vi "TD VI.vi"() -> ()   [LabVIEW 2016]
panel:
  out "Desvio Padrão":dbl
  out "Média":dbl
  out "Vetor de amostras":dbl[](array[numeric])
  out "Waveform Chart":dbl(graph)
  out "Amostra":dbl
  out "error out":errorcluster
  in  "acende botão":bool
  in  "Stop Button":bool
  in  "Send":bool
  in  "VISA resource name":refnum<visa-resource-name>
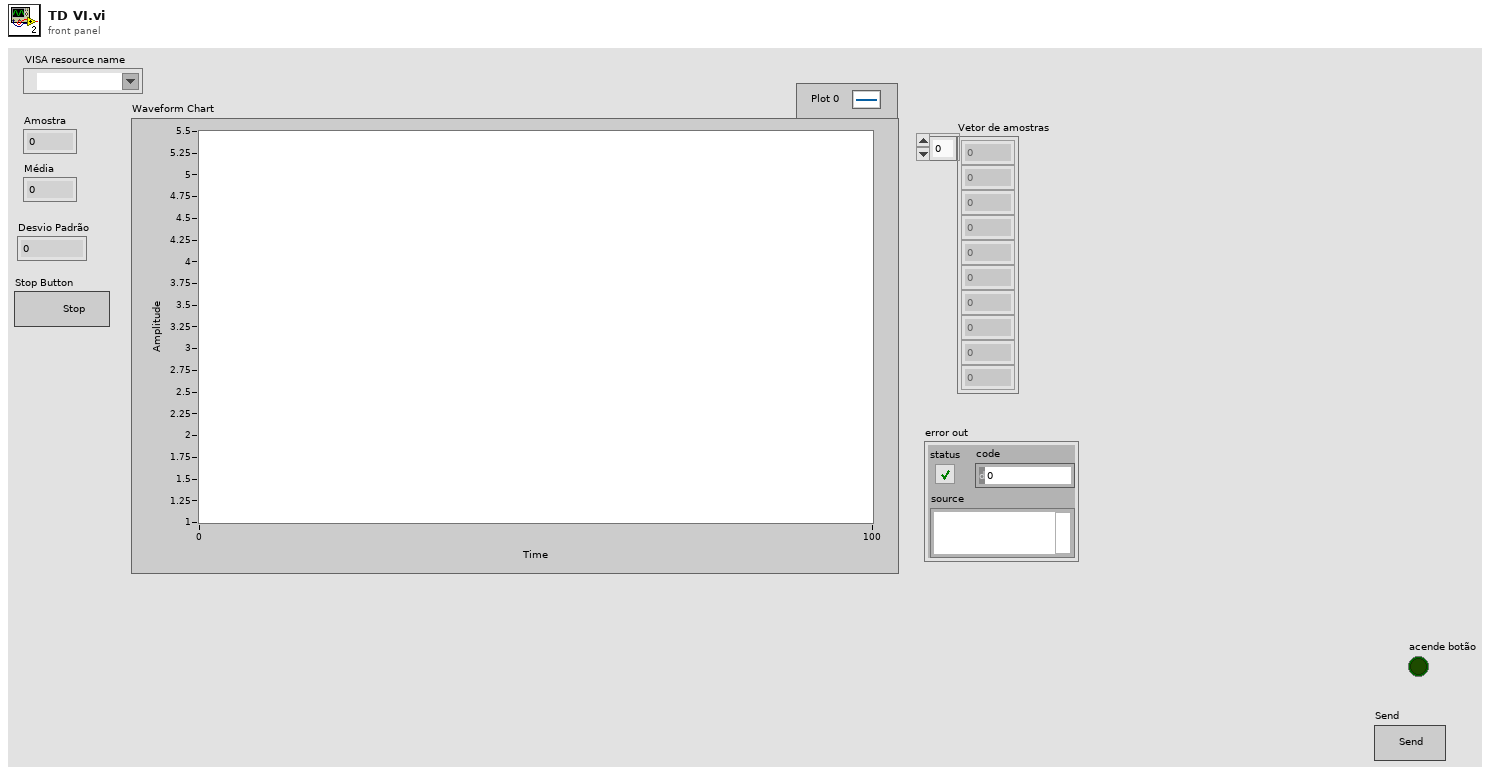
[diagram p1: front panel]
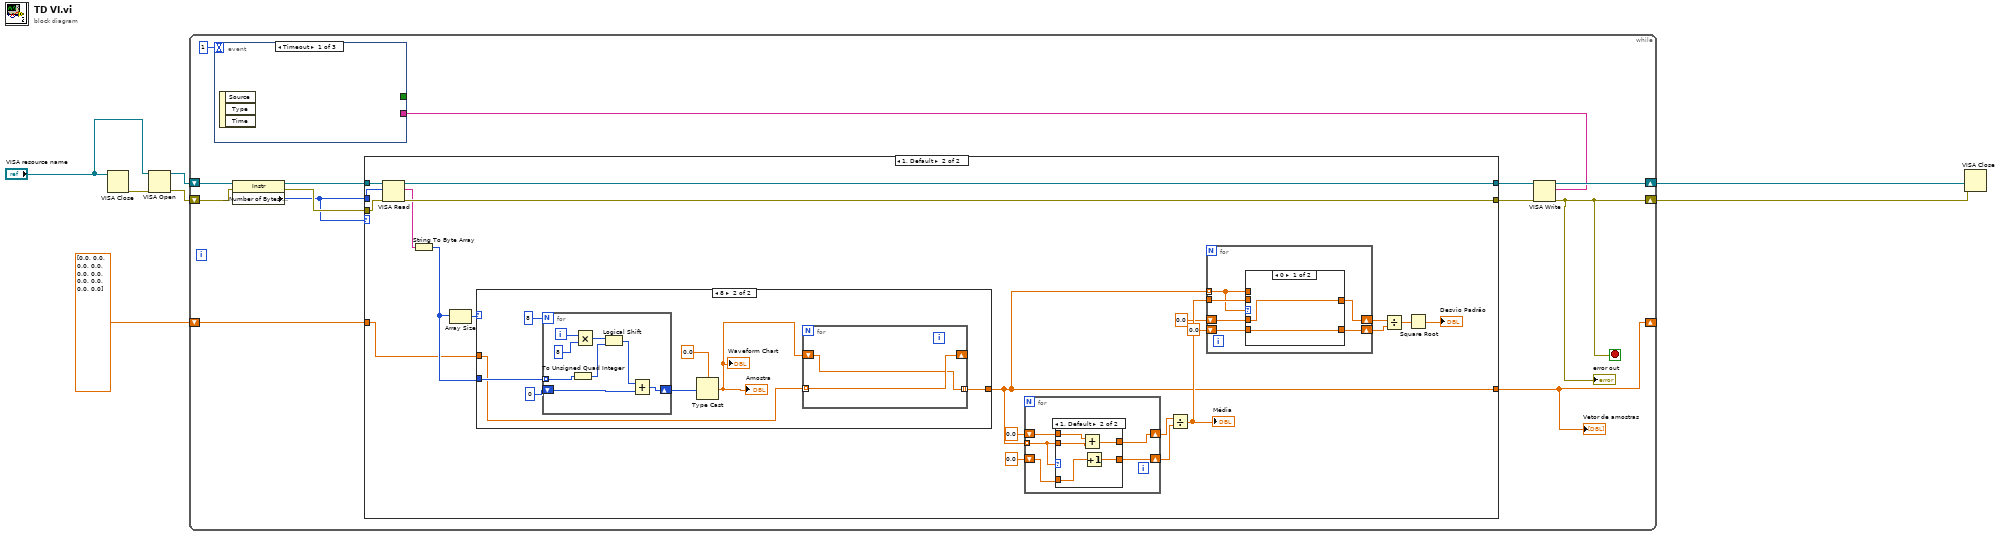
[diagram p0: block diagram]
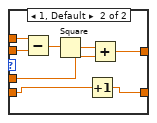
[diagram p4: hidden frame]
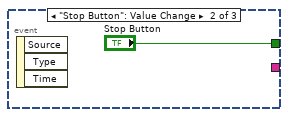
[diagram p6: hidden frame]
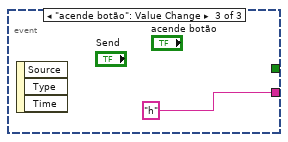
[diagram p7: hidden frame]
diagram:
  n1 = VISA Close(VISA resource name="VISA resource name") -> (error out=w4:errorcluster)  [unwired: 1 in]
  n2 = VISA Open(error in (no error)=w4, VISA resource name="VISA resource name") -> (VISA resource name=w3:refnum<visa-resource-name>, error out=w2:errorcluster)  [unwired: 3 in]
  n3 = while {
    shift-right: [w20] -> w6
    shift-left: w3 -> [w16]
    shift-right: [w10] -> w7
    shift-left: w2 -> [w14]
    shift-right: [w8] -> _
    shift-left: dbl[] [0.0, 0.0, 0.0, 0.0, 0.0, 0.0, 0.0, 0.0, 0.0, 0.0] -> [w9]
    stop <- w10 stop-if-true
    n4 = event shown="[0] Timeout" {
      selector: _ -> [_ _ _]
      dyn-events: _ -> [_ _ _]
      timeout: 1 -> [_ _ _]
      tunnel: [_ "Stop Button" _] -> _
      tunnel: [_ _ "h" ("write buffer")] -> w17
      event Timeout {
        n5 = event-data() -> ()  [unwired: 1 in, 3 out]
      }
      event "Stop Button": Value Change {
        n6 = event-data() -> ()  [unwired: 1 in, 3 out]
      }
      event "acende botão": Value Change {
        n7 = event-data() -> ()  [unwired: 1 in, 3 out]
      }
    }
    n8 = property class="Instr"(reference=w16, error in=w14) -> (reference out=w15:refnum<visa-resource-name>, error out=w13:errorcluster, "Serial Settings:Number of Bytes at Serial Port"=w11:u32)
    n9 = case shown="1, Default" w11 {
      tunnel: [w22 w44] -> w19
      tunnel: [w23 w43] -> w18
      tunnel: w15 -> [w23 w42]
      tunnel: w11 -> [_ w41]
      tunnel: w13 -> [w22 w40]
      tunnel: w9 -> [w21 w36]
      tunnel: [w21 w30] -> w8
      frame 0 {
      }
      frame 1, Default {
        n10 = VISA Read(VISA resource name=w42, byte count=w41, error in (no error)=w40) -> (VISA resource name out=w43:refnum<visa-resource-name>, read buffer=w39:string, error out=w44:errorcluster)  [unwired: 1 out]
        n11 = String To Byte Array(string=w39) -> (unsigned byte array=w37:u8[])
        n12 = Array Size(array=w37) -> (size(s)=w38:i32)
        n13 = case shown="8" w38 {
          tunnel: w37 -> [_ w80]
          tunnel: w36 -> [w73 w76]
          tunnel: [w73 w75] -> w30
          frame 0, Default {
          }
          frame 8 {
            n14 = for {
              N: 8 -> [_]
              tunnel: w80 -> [w88] mode=indexing
              shift-right: [w85] -> w78
              shift-left: u64 0 -> [w84]
              i -> [w91]
              n15 = To Unsigned Quad Integer(1:w88) -> (0:w87:u64)
              n16 = Multiply(x=w91, y=8) -> (x*y=w89:i32)
              n17 = Logical Shift(y=w89, x=w87) -> (x << y=w86:u64)
              n18 = Add(x=w86, y=w84) -> (x+y=w85:u64)
            }
            n19 = Type Cast(type=0.0, x=w78) -> (*(type *) &x=w74:dbl)
            "Amostra" <- w74
            "Waveform Chart" <- w74
            n20 = for {
              tunnel: w76 -> [w83] mode=indexing
              tunnel: [w82] -> w75 mode=indexing
              shift-right: [w83] -> _
              shift-left: w74 -> [w82]
            }
          }
        }
        n21 = for {
          tunnel: w30 -> [w47] mode=indexing
          shift-right: [w48] -> w29
          shift-left: 0.0 -> [w49]
          shift-right: [w46] -> w27
          shift-left: 0.0 -> [w45]
          n22 = case shown="1, Default" w47 {
            tunnel: w49 -> [w51 w56]
            tunnel: [w51 w55] -> w48
            tunnel: w47 -> [_ w54]
            tunnel: [w50 w52] -> w46
            tunnel: w45 -> [w50 w53]
            frame 0 {
            }
            frame 1, Default {
              n23 = Add(x=w56, y=w54) -> (x+y=w55:dbl)
              n24 = Increment(x=w53) -> (x+1=w52:dbl)
            }
          }
        }
        n25 = Divide(x=w29, y=w27) -> (x/y=w35:dbl)
        "Média" <- w35
        n26 = for {
          tunnel: w30 -> [w59] mode=indexing
          tunnel: w35 -> [w62]
          shift-right: [w61] -> w33
          shift-left: 0.0 -> [w60]
          shift-right: [w58] -> w24
          shift-left: 0.0 -> [w57]
          n27 = case shown="0" w59 {
            tunnel: w59 -> [_ w72]
            tunnel: w62 -> [_ w71]
            tunnel: [w63 w70] -> w61
            tunnel: w60 -> [w63 w69]
            tunnel: [w64 w66] -> w58
            tunnel: w57 -> [w64 w65]
            frame 0 {
            }
            frame 1, Default {
              n28 = Subtract(x=w72, y=w71) -> (x-y=w67:dbl)
              n29 = Square(x=w67) -> (x^2=w68:dbl)
              n30 = Increment(x=w65) -> (x+1=w66:dbl)
              n31 = Add(x=w68, y=w69) -> (x+y=w70:dbl)
            }
          }
        }
        n32 = Divide(x=w33, y=w24) -> (x/y=w32:dbl)
        n33 = Square Root(x=w32) -> (sqrt(x)=→"Desvio Padrão":dbl)
      }
    }
    "Vetor de amostras" <- w8
    n34 = VISA Write(VISA resource name=w18, write buffer=w17, error in (no error)=w19) -> (VISA resource name out=w20:refnum<visa-resource-name>, error out=w10:errorcluster)  [unwired: 1 out]
    "error out" <- w10
  }
  n35 = VISA Close(VISA resource name=w6, error in (no error)=w7) -> ()  [unwired: 1 out]
